vi "remainin time.vi"() -> ()   [LabVIEW 2025]
uses:
  kernel32.dll
panel:
  in  "Remaining Time":dbl min=0.0 max=180000.0 step=0.0001 format="%<%H:%M:%S>t"
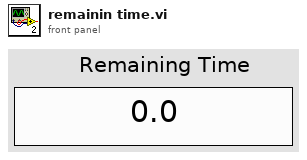
[diagram p1: front panel]
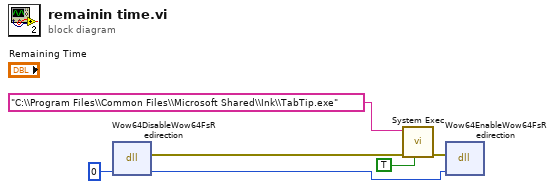
[diagram p0: block diagram]
diagram:
  n1 = dll-call lib="kernel32.dll" fn="Wow64DisableWow64FsRedirection"("OldValue"=0) -> (error out=w3:errorcluster, "OldValue"=w5:i32)  [unwired: 4 in, 1 out]
  n2 = call <vilib>:"System Exec.vi"("run minimized? (F)"=TRUE, "error in (no error)"=w3, "command line"="C:\\Program Files\\Common Files\\Microsoft Shared\\Ink\\TabTip.exe") -> ("error out"=w4:errorcluster)  [unwired: 5 in, 3 out]
  n3 = dll-call lib="kernel32.dll" fn="Wow64EnableWow64FsRedirection"(error in=w4, "OldValue"=w5) -> ()  [unwired: 4 in, 2 out]
